vi "myRIO_BRig_RT_dataExp_Cue1Param_CueType_NS.vi"() -> (2 "output_Cue1Param_CueType_NS":i32)   [LabVIEW 2014]
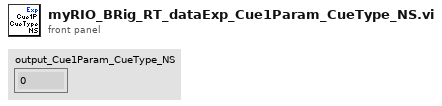
[diagram p1: front panel]
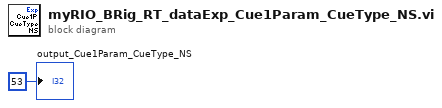
[diagram p0: block diagram]
diagram:
  "output_Cue1Param_CueType_NS" <- 53 ("output_iBlock")
